vi "DataMatrix AutoDetect Parameters.vi"(7 "_Barcode Type":u16(ring) caption="Barcode Type" items=["Data Matrix", "PDF417", "QR Code"], 8 "error in (no error)":errorcluster, 10 "ROI Descriptor":T20 {"Contours"."Type" items=["No Selection", "Point", "Line", "Rectangle", "Oval", "Polygon", "Free", "Annulus", "Unused2", "Unused3", "Broken Line", "Free Hand Line", "Rotated Rectangle"]}, 11 "Image":T17) -> (0 "error out":errorcluster, 2 "QR Code Auto Detect Values":T8={"QR Search Options"={"Rotation Mode"=enum."Unlimited", "Skip Location?"=FALSE, "Edge Threshold"=30, "Demodulation Mode"=-2, "Cell Sample Size"=-2, "Cell Filter Mode"=-2, "Skew Degrees Allowed"=5}, "QR Description Options"={"Matrix Size (cells)"=0, "Barcode Polarity"=-2, "Mirror Mode"=-2, "QR Model"=0}, "QR Code Cell Size (pixels)"={"Minimum Size"=3, "Maximum Size"=7}} {"QR Description Options"."Mirror Mode" items=["Auto-detect"=-2, "Normal"=0, "Mirrored"=1]; "QR Description Options"."Matrix Size (cells)" items=["Auto-detect"=0, "11x11 - Version 1 (Micro QR Only)"=11, "13x13 - Version 2 (Micro QR Only)"=13, "15x15 - Version 3 (Micro QR Only)"=15, "17x17 - Version 4 (Micro QR Only)"=17, "21x21 - Version 1"=21, "25x25 - Version 2"=25, "29x29 - Version 3"=29, "33x33 - Version 4"=33, "37x37 - Version 5"=37, "41x41 - Version 6"=41, "45x45 - Version 7"=45, "49x49 - Version 8"=49, "53x53 - Version 9"=53, "57x57 - Version 10"=57, "61x61 - Version 11"=61, "65x65 - Version 12"=65, "69x69 - Version 13"=69, "73x73 - Version 14"=73, "77x77 - Version 15"=77, "81x81 - Version 16"=81, "85x85 - Version 17"=85, "89x89 - Version 18"=89, "93x93 - Version 19"=93, "97x97 - Version 20"=97, "101x101 - Version 21"=101, "105x105 - Version 22"=105, "109x109 - Version 23"=109, "113x113 - Version 24"=113, "117x117 - Version 25"=117, "121x121 - Version 26"=121, "125x125 - Version 27"=125, "129x129 - Version 28"=129, "133x133 - Version 29"=133, "137x137 - Version 30"=137, "141x141 - Version 31"=141, "145x145 - Version 32"=145, "149x149 - Version 33"=149, "153x153 - Version 34"=153, "157x157 - Version 35"=157, "161x161 - Version 36"=161, "165x165 - Version 37"=165, "169x169 -  Version 38"=169, "173x173 - Version 39"=173, "177x177 - Version 40"=177]; "QR Description Options"."QR Model" items=["Auto-detect", "Micro", "Model 1", "Model 2"]; "QR Description Options"."Barcode Polarity" items=["Auto-detect"=-2, "Black on White"=0, "White on Black"=1]; "QR Search Options"."Cell Filter Mode" items=["Auto-detect"=-2, "Average"=0, "Median"=1, "Central Average"=2, "High Average"=3, "Low Average"=4, "Very High Average"=5, "Very Low Average"=6, "All Filters"=8]; "QR Search Options"."Cell Sample Size" items=["Auto-detect"=-2, "1x1"=1, "2x2"=2, "3x3"=3, "4x4"=4, "5x5"=5, "6x6"=6, "7x7"=7]; "QR Search Options"."Demodulation Mode" items=["Auto-detect"=-2, "Histogram"=0, "Local Contrast"=1, "Combination"=2, "All"=3]}, 3 "Data Matrix Auto Detect Values Out":T16={"Data Matrix Description Options"={"Aspect Ratio"=0.0, "Rows"=0, "Columns"=0, "Rectangle"=FALSE, "ECC"=-2, "Barcode Polarity"=-2, "Cell Fill Percentage"=-2, "Minimum Border Integrity %"=80.0, "Mirror Mode"=-2}, "Data Matrix Search Options"={"Rotation Mode"=enum."Unlimited", "Skip Location?"=FALSE, "Edge Threshold"=30, "Demodulation Mode"=-2, "Cell Sample Size"=-2, "Cell Filter Mode"=-2, "Skew Degrees Allowed"=5, "Maximum Iterations"=500, "Initial Search Vector Width"=5}, "Data Matrix Size Options"={"Data Matrix Size"={"Minimum Size"=0, "Maximum Size"=0}, "Quiet Zone Width"=10}, "Advanced Options"=[]} {"Advanced Options"."Value" format="%.2f"; "Data Matrix Search Options"."Cell Filter Mode" items=["Auto-detect"=-2, "Average"=0, "Median"=1, "Central Average"=2, "High Average"=3, "Low Average"=4, "Very High Average"=5, "Very Low Average"=6, "All Filters"=8]; "Data Matrix Search Options"."Cell Sample Size" items=["Auto-detect"=-2, "1x1"=1, "2x2"=2, "3x3"=3, "4x4"=4, "5x5"=5, "6x6"=6, "7x7"=7]; "Data Matrix Search Options"."Demodulation Mode" items=["Auto-detect"=-2, "Histogram"=0, "Local Contrast"=1, "Combination"=2, "All"=3]; "Data Matrix Description Options"."Mirror Mode" items=["Auto-detect"=-2, "Normal"=0, "Mirrored"=1]; "Data Matrix Description Options"."ECC" items=["Auto-detect"=-2, "ECC 000"=0, "ECC 050"=50, "ECC 080"=80, "ECC 100"=100, "ECC 140"=140, "ECC 000-140"=190, "ECC 200"=200]; "Data Matrix Description Options"."Minimum Border Integrity %" format="%.2f"; "Data Matrix Description Options"."Aspect Ratio" format="%.2f"; "Data Matrix Description Options"."Cell Fill Percentage" items=["Auto-detect"=-2, "< 30%"=0, ">= 30%"=1]; "Data Matrix Description Options"."Barcode Polarity" items=["Auto-detect"=-2, "Black on White"=0, "White on Black"=1]})   [LabVIEW 2015]
uses:
  <vilib>/vision/Instrument.llb/Data Matrix Description Options.ctl
  <vilib>/vision/Instrument.llb/ECC Type.ctl
  <vilib>/vision/Instrument.llb/Data Matrix Polarity.ctl
  <vilib>/vision/Instrument.llb/Cell Fill Percentage.ctl
  <vilib>/vision/Instrument.llb/Data Matrix Mirror.ctl
  <vilib>/vision/Instrument.llb/Data Matrix Search Options.ctl
  <vilib>/vision/Instrument.llb/Demodulation Mode.ctl
  <vilib>/vision/Instrument.llb/Cell Sample Size.ctl
  <vilib>/vision/Instrument.llb/Cell Filter Mode.ctl
  <vilib>/vision/Instrument.llb/Data Matrix Size Options.ctl
  <vilib>/vision/Instrument.llb/Data Matrix Advanced Options.ctl
  <vilib>/vision/Instrument.llb/QR Code Search Options.ctl
  <vilib>/vision/Instrument.llb/QR Code Description Options.ctl
  <vilib>/vision/Instrument.llb/QR Code Model Type.ctl
  <vilib>/vision/Image Controls.llb/IMAQ Image.ctl
  <vilib>/vision/NI_Vision_Development_Module.lvlib
panel:
  in  "QR Code Auto Detect Values":T18(array[cluster])=[{"QR Search Options"={"Rotation Mode"=enum."Unlimited", "Skip Location?"=FALSE, "Edge Threshold"=30, "Demodulation Mode"=-2, "Cell Sample Size"=-2, "Cell Filter Mode"=2, "Skew Degrees Allowed"=5}, "QR Description Options"={"Matrix Size (cells)"=0, "Barcode Polarity"=-2, "Mirror Mode"=-2, "QR Model"=0}, "QR Code Cell Size (pixels)"={"Minimum Size"=3, "Maximum Size"=15}}, {"QR Search Options"={"Rotation Mode"=enum."Unlimited", "Skip Location?"=FALSE, "Edge Threshold"=15, "Demodulation Mode"=-2, "Cell Sample Size"=-2, "Cell Filter Mode"=2, "Skew Degrees Allowed"=15}, "QR Description Options"={"Matrix Size (cells)"=0, "Barcode Polarity"=-2, "Mirror Mode"=0, "QR Model"=0}, "QR Code Cell Size (pixels)"={"Minimum Size"=3, "Maximum Size"=15}}, {"QR Search Options"={"Rotation Mode"=enum."Unlimited", "Skip Location?"=FALSE, "Edge Threshold"=15, "Demodulation Mode"=-2, "Cell Sample Size"=-2, "Cell Filter Mode"=2, "Skew Degrees Allowed"=15}, "QR Description Options"={"Matrix Size (cells)"=0, "Barcode Polarity"=-2, "Mirror Mode"=-2, "QR Model"=0}, "QR Code Cell Size (pixels)"={"Minimum Size"=3, "Maximum Size"=15}}, {"QR Search Options"={"Rotation Mode"=enum."Unlimited", "Skip Location?"=FALSE, "Edge Threshold"=5, "Demodulation Mode"=-2, "Cell Sample Size"=-2, "Cell Filter Mode"=2, "Skew Degrees Allowed"=15}, "QR Description Options"={"Matrix Size (cells)"=0, "Barcode Polarity"=-2, "Mirror Mode"=-2, "QR Model"=0}, "QR Code Cell Size (pixels)"={"Minimum Size"=3, "Maximum Size"=15}}, {"QR Search Options"={"Rotation Mode"=enum."Unlimited", "Skip Location?"=FALSE, "Edge Threshold"=30, "Demodulation Mode"=-2, "Cell Sample Size"=-2, "Cell Filter Mode"=-2, "Skew Degrees Allowed"=3}, "QR Description Options"={"Matrix Size (cells)"=0, "Barcode Polarity"=-2, "Mirror Mode"=-2, "QR Model"=0}, "QR Code Cell Size (pixels)"={"Minimum Size"=3, "Maximum Size"=15}}, {"QR Search Options"={"Rotation Mode"=enum."Unlimited", "Skip Location?"=FALSE, "Edge Threshold"=5, "Demodulation Mode"=-2, "Cell Sample Size"=-2, "Cell Filter Mode"=2, "Skew Degrees Allowed"=5}, "QR Description Options"={"Matrix Size (cells)"=0, "Barcode Polarity"=-2, "Mirror Mode"=-2, "QR Model"=0}, "QR Code Cell Size (pixels)"={"Minimum Size"=3, "Maximum Size"=15}}, {"QR Search Options"={"Rotation Mode"=enum."Unlimited", "Skip Location?"=FALSE, "Edge Threshold"=20, "Demodulation Mode"=-2, "Cell Sample Size"=-2, "Cell Filter Mode"=2, "Skew Degrees Allowed"=5}, "QR Description Options"={"Matrix Size (cells)"=0, "Barcode Polarity"=-2, "Mirror Mode"=-2, "QR Model"=0}, "QR Code Cell Size (pixels)"={"Minimum Size"=3, "Maximum Size"=15}}, {"QR Search Options"={"Rotation Mode"=enum."Unlimited", "Skip Location?"=FALSE, "Edge Threshold"=50, "Demodulation Mode"=-2, "Cell Sample Size"=-2, "Cell Filter Mode"=2, "Skew Degrees Allowed"=5}, "QR Description Options"={"Matrix Size (cells)"=0, "Barcode Polarity"=-2, "Mirror Mode"=-2, "QR Model"=0}, "QR Code Cell Size (pixels)"={"Minimum Size"=3, "Maximum Size"=15}}] {"QR Description Options"."Mirror Mode" items=["Auto-detect"=-2, "Normal"=0, "Mirrored"=1]; "QR Description Options"."Matrix Size (cells)" items=["Auto-detect"=0, "11x11 - Version 1 (Micro QR Only)"=11, "13x13 - Version 2 (Micro QR Only)"=13, "15x15 - Version 3 (Micro QR Only)"=15, "17x17 - Version 4 (Micro QR Only)"=17, "21x21 - Version 1"=21, "25x25 - Version 2"=25, "29x29 - Version 3"=29, "33x33 - Version 4"=33, "37x37 - Version 5"=37, "41x41 - Version 6"=41, "45x45 - Version 7"=45, "49x49 - Version 8"=49, "53x53 - Version 9"=53, "57x57 - Version 10"=57, "61x61 - Version 11"=61, "65x65 - Version 12"=65, "69x69 - Version 13"=69, "73x73 - Version 14"=73, "77x77 - Version 15"=77, "81x81 - Version 16"=81, "85x85 - Version 17"=85, "89x89 - Version 18"=89, "93x93 - Version 19"=93, "97x97 - Version 20"=97, "101x101 - Version 21"=101, "105x105 - Version 22"=105, "109x109 - Version 23"=109, "113x113 - Version 24"=113, "117x117 - Version 25"=117, "121x121 - Version 26"=121, "125x125 - Version 27"=125, "129x129 - Version 28"=129, "133x133 - Version 29"=133, "137x137 - Version 30"=137, "141x141 - Version 31"=141, "145x145 - Version 32"=145, "149x149 - Version 33"=149, "153x153 - Version 34"=153, "157x157 - Version 35"=157, "161x161 - Version 36"=161, "165x165 - Version 37"=165, "169x169 -  Version 38"=169, "173x173 - Version 39"=173, "177x177 - Version 40"=177]; "QR Description Options"."QR Model" items=["Auto-detect", "Micro", "Model 1", "Model 2"]; "QR Description Options"."Barcode Polarity" items=["Auto-detect"=-2, "Black on White"=0, "White on Black"=1]; "QR Search Options"."Cell Filter Mode" items=["Auto-detect"=-2, "Average"=0, "Median"=1, "Central Average"=2, "High Average"=3, "Low Average"=4, "Very High Average"=5, "Very Low Average"=6, "All Filters"=8]; "QR Search Options"."Cell Sample Size" items=["Auto-detect"=-2, "1x1"=1, "2x2"=2, "3x3"=3, "4x4"=4, "5x5"=5, "6x6"=6, "7x7"=7]; "QR Search Options"."Demodulation Mode" items=["Auto-detect"=-2, "Histogram"=0, "Local Contrast"=1, "Combination"=2, "All"=3]}
  in  "Data Matrix Auto Detect Values":T19(array[cluster])=[{"Data Matrix Description Options"={"Aspect Ratio"=0.0, "Rows"=0, "Columns"=0, "Rectangle"=FALSE, "ECC"=-2, "Barcode Polarity"=-2, "Cell Fill Percentage"=-2, "Minimum Border Integrity %"=80.0, "Mirror Mode"=-2}, "Data Matrix Search Options"={"Rotation Mode"=enum."Unlimited", "Skip Location?"=FALSE, "Edge Threshold"=30, "Demodulation Mode"=-2, "Cell Sample Size"=-2, "Cell Filter Mode"=2, "Skew Degrees Allowed"=5, "Maximum Iterations"=100, "Initial Search Vector Width"=5}, "Data Matrix Size Options"={"Data Matrix Size"={"Minimum Size"=0, "Maximum Size"=0}, "Quiet Zone Width"=0}, "Advanced Options"=[]}, {"Data Matrix Description Options"={"Aspect Ratio"=0.0, "Rows"=0, "Columns"=0, "Rectangle"=FALSE, "ECC"=-2, "Barcode Polarity"=-2, "Cell Fill Percentage"=-2, "Minimum Border Integrity %"=80.0, "Mirror Mode"=-2}, "Data Matrix Search Options"={"Rotation Mode"=enum."Unlimited", "Skip Location?"=FALSE, "Edge Threshold"=30, "Demodulation Mode"=-2, "Cell Sample Size"=-2, "Cell Filter Mode"=2, "Skew Degrees Allowed"=5, "Maximum Iterations"=100, "Initial Search Vector Width"=15}, "Data Matrix Size Options"={"Data Matrix Size"={"Minimum Size"=0, "Maximum Size"=0}, "Quiet Zone Width"=0}, "Advanced Options"=[{"Option"=enum."Line Detection", " Value"=1.0}]}, {"Data Matrix Description Options"={"Aspect Ratio"=0.0, "Rows"=0, "Columns"=0, "Rectangle"=FALSE, "ECC"=-2, "Barcode Polarity"=-2, "Cell Fill Percentage"=-2, "Minimum Border Integrity %"=75.0, "Mirror Mode"=0}, "Data Matrix Search Options"={"Rotation Mode"=enum."Unlimited", "Skip Location?"=FALSE, "Edge Threshold"=15, "Demodulation Mode"=-2, "Cell Sample Size"=-2, "Cell Filter Mode"=2, "Skew Degrees Allowed"=15, "Maximum Iterations"=500, "Initial Search Vector Width"=15}, "Data Matrix Size Options"={"Data Matrix Size"={"Minimum Size"=0, "Maximum Size"=0}, "Quiet Zone Width"=0}, "Advanced Options"=[]}, {"Data Matrix Description Options"={"Aspect Ratio"=0.0, "Rows"=0, "Columns"=0, "Rectangle"=FALSE, "ECC"=-2, "Barcode Polarity"=-2, "Cell Fill Percentage"=-2, "Minimum Border Integrity %"=75.0, "Mirror Mode"=-2}, "Data Matrix Search Options"={"Rotation Mode"=enum."Unlimited", "Skip Location?"=FALSE, "Edge Threshold"=15, "Demodulation Mode"=-2, "Cell Sample Size"=-2, "Cell Filter Mode"=2, "Skew Degrees Allowed"=15, "Maximum Iterations"=100, "Initial Search Vector Width"=15}, "Data Matrix Size Options"={"Data Matrix Size"={"Minimum Size"=0, "Maximum Size"=0}, "Quiet Zone Width"=0}, "Advanced Options"=[{"Option"=enum."Line Detection", " Value"=1.0}, {"Option"=enum."HighLight Filter", " Value"=0.0}]}, {"Data Matrix Description Options"={"Aspect Ratio"=0.0, "Rows"=0, "Columns"=0, "Rectangle"=FALSE, "ECC"=-2, "Barcode Polarity"=-2, "Cell Fill Percentage"=-2, "Minimum Border Integrity %"=75.0, "Mirror Mode"=-2}, "Data Matrix Search Options"={"Rotation Mode"=enum."Unlimited", "Skip Location?"=FALSE, "Edge Threshold"=5, "Demodulation Mode"=-2, "Cell Sample Size"=-2, "Cell Filter Mode"=2, "Skew Degrees Allowed"=15, "Maximum Iterations"=100, "Initial Search Vector Width"=15}, "Data Matrix Size Options"={"Data Matrix Size"={"Minimum Size"=0, "Maximum Size"=0}, "Quiet Zone Width"=0}, "Advanced Options"=[{"Option"=enum."Line Detection", " Value"=0.0}, {"Option"=enum."HighLight Filter", " Value"=0.0}]}, {"Data Matrix Description Options"={"Aspect Ratio"=0.0, "Rows"=0, "Columns"=0, "Rectangle"=FALSE, "ECC"=-2, "Barcode Polarity"=-2, "Cell Fill Percentage"=-2, "Minimum Border Integrity %"=75.0, "Mirror Mode"=-2}, "Data Matrix Search Options"={"Rotation Mode"=enum."Unlimited", "Skip Location?"=FALSE, "Edge Threshold"=5, "Demodulation Mode"=-2, "Cell Sample Size"=-2, "Cell Filter Mode"=2, "Skew Degrees Allowed"=15, "Maximum Iterations"=100, "Initial Search Vector Width"=15}, "Data Matrix Size Options"={"Data Matrix Size"={"Minimum Size"=0, "Maximum Size"=0}, "Quiet Zone Width"=0}, "Advanced Options"=[{"Option"=enum."Line Detection", " Value"=1.0}, {"Option"=enum."HighLight Filter", " Value"=1.0}]}, {"Data Matrix Description Options"={"Aspect Ratio"=0.0, "Rows"=0, "Columns"=0, "Rectangle"=FALSE, "ECC"=-2, "Barcode Polarity"=-2, "Cell Fill Percentage"=-2, "Minimum Border Integrity %"=80.0, "Mirror Mode"=-2}, "Data Matrix Search Options"={"Rotation Mode"=enum."Unlimited", "Skip Location?"=FALSE, "Edge Threshold"=30, "Demodulation Mode"=-2, "Cell Sample Size"=-2, "Cell Filter Mode"=-2, "Skew Degrees Allowed"=3, "Maximum Iterations"=100, "Initial Search Vector Width"=5}, "Data Matrix Size Options"={"Data Matrix Size"={"Minimum Size"=75, "Maximum Size"=175}, "Quiet Zone Width"=0}, "Advanced Options"=[{"Option"=enum."Line Detection", " Value"=0.0}, {"Option"=enum."HighLight Filter", " Value"=0.0}]}, {"Data Matrix Description Options"={"Aspect Ratio"=0.0, "Rows"=0, "Columns"=0, "Rectangle"=FALSE, "ECC"=-2, "Barcode Polarity"=-2, "Cell Fill Percentage"=-2, "Minimum Border Integrity %"=80.0, "Mirror Mode"=-2}, "Data Matrix Search Options"={"Rotation Mode"=enum."Unlimited", "Skip Location?"=FALSE, "Edge Threshold"=5, "Demodulation Mode"=-2, "Cell Sample Size"=-2, "Cell Filter Mode"=2, "Skew Degrees Allowed"=5, "Maximum Iterations"=100, "Initial Search Vector Width"=5}, "Data Matrix Size Options"={"Data Matrix Size"={"Minimum Size"=75, "Maximum Size"=175}, "Quiet Zone Width"=0}, "Advanced Options"=[]}, {"Data Matrix Description Options"={"Aspect Ratio"=0.0, "Rows"=0, "Columns"=0, "Rectangle"=FALSE, "ECC"=-2, "Barcode Polarity"=-2, "Cell Fill Percentage"=-2, "Minimum Border Integrity %"=80.0, "Mirror Mode"=-2}, "Data Matrix Search Options"={"Rotation Mode"=enum."Unlimited", "Skip Location?"=FALSE, "Edge Threshold"=20, "Demodulation Mode"=-2, "Cell Sample Size"=-2, "Cell Filter Mode"=2, "Skew Degrees Allowed"=5, "Maximum Iterations"=100, "Initial Search Vector Width"=5}, "Data Matrix Size Options"={"Data Matrix Size"={"Minimum Size"=0, "Maximum Size"=0}, "Quiet Zone Width"=0}, "Advanced Options"=[{"Option"=enum."Refine Bounding Box", " Value"=0.0}]}, {"Data Matrix Description Options"={"Aspect Ratio"=0.0, "Rows"=0, "Columns"=0, "Rectangle"=FALSE, "ECC"=-2, "Barcode Polarity"=-2, "Cell Fill Percentage"=-2, "Minimum Border Integrity %"=80.0, "Mirror Mode"=-2}, "Data Matrix Search Options"={"Rotation Mode"=enum."Unlimited", "Skip Location?"=FALSE, "Edge Threshold"=20, "Demodulation Mode"=-2, "Cell Sample Size"=-2, "Cell Filter Mode"=2, "Skew Degrees Allowed"=5, "Maximum Iterations"=50, "Initial Search Vector Width"=15}, "Data Matrix Size Options"={"Data Matrix Size"={"Minimum Size"=0, "Maximum Size"=0}, "Quiet Zone Width"=0}, "Advanced Options"=[{"Option"=enum."Line Detection", " Value"=1.0}]}, {"Data Matrix Description Options"={"Aspect Ratio"=0.0, "Rows"=0, "Columns"=0, "Rectangle"=FALSE, "ECC"=-2, "Barcode Polarity"=-2, "Cell Fill Percentage"=-2, "Minimum Border Integrity %"=80.0, "Mirror Mode"=-2}, "Data Matrix Search Options"={"Rotation Mode"=enum."Unlimited", "Skip Location?"=FALSE, "Edge Threshold"=50, "Demodulation Mode"=-2, "Cell Sample Size"=-2, "Cell Filter Mode"=2, "Skew Degrees Allowed"=5, "Maximum Iterations"=50, "Initial Search Vector Width"=5}, "Data Matrix Size Options"={"Data Matrix Size"={"Minimum Size"=50, "Maximum Size"=300}, "Quiet Zone Width"=0}, "Advanced Options"=[{"Option"=enum."Line Detection", " Value"=0.0}]}, {"Data Matrix Description Options"={"Aspect Ratio"=0.0, "Rows"=0, "Columns"=0, "Rectangle"=FALSE, "ECC"=-2, "Barcode Polarity"=-2, "Cell Fill Percentage"=-2, "Minimum Border Integrity %"=80.0, "Mirror Mode"=-2}, "Data Matrix Search Options"={"Rotation Mode"=enum."Unlimited", "Skip Location?"=FALSE, "Edge Threshold"=30, "Demodulation Mode"=-2, "Cell Sample Size"=-2, "Cell Filter Mode"=2, "Skew Degrees Allowed"=5, "Maximum Iterations"=50, "Initial Search Vector Width"=5}, "Data Matrix Size Options"={"Data Matrix Size"={"Minimum Size"=175, "Maximum Size"=350}, "Quiet Zone Width"=0}, "Advanced Options"=[{"Option"=enum."Refine Bounding Box", " Value"=1.0}]}, {"Data Matrix Description Options"={"Aspect Ratio"=0.0, "Rows"=0, "Columns"=0, "Rectangle"=TRUE, "ECC"=-2, "Barcode Polarity"=-2, "Cell Fill Percentage"=-2, "Minimum Border Integrity %"=80.0, "Mirror Mode"=-2}, "Data Matrix Search Options"={"Rotation Mode"=enum."Unlimited", "Skip Location?"=FALSE, "Edge Threshold"=30, "Demodulation Mode"=-2, "Cell Sample Size"=-2, "Cell Filter Mode"=2, "Skew Degrees Allowed"=5, "Maximum Iterations"=30, "Initial Search Vector Width"=5}, "Data Matrix Size Options"={"Data Matrix Size"={"Minimum Size"=0, "Maximum Size"=0}, "Quiet Zone Width"=0}, "Advanced Options"=[{"Option"=enum."Line Detection", " Value"=1.0}]}] {"Advanced Options"."Value" format="%.2f"; "Data Matrix Search Options"."Cell Filter Mode" items=["Auto-detect"=-2, "Average"=0, "Median"=1, "Central Average"=2, "High Average"=3, "Low Average"=4, "Very High Average"=5, "Very Low Average"=6, "All Filters"=8]; "Data Matrix Search Options"."Cell Sample Size" items=["Auto-detect"=-2, "1x1"=1, "2x2"=2, "3x3"=3, "4x4"=4, "5x5"=5, "6x6"=6, "7x7"=7]; "Data Matrix Search Options"."Demodulation Mode" items=["Auto-detect"=-2, "Histogram"=0, "Local Contrast"=1, "Combination"=2, "All"=3]; "Data Matrix Description Options"."Mirror Mode" items=["Auto-detect"=-2, "Normal"=0, "Mirrored"=1]; "Data Matrix Description Options"."ECC" items=["Auto-detect"=-2, "ECC 000"=0, "ECC 050"=50, "ECC 080"=80, "ECC 100"=100, "ECC 140"=140, "ECC 000-140"=190, "ECC 200"=200]; "Data Matrix Description Options"."Minimum Border Integrity %" format="%.2f"; "Data Matrix Description Options"."Aspect Ratio" format="%.2f"; "Data Matrix Description Options"."Cell Fill Percentage" items=["Auto-detect"=-2, "< 30%"=0, ">= 30%"=1]; "Data Matrix Description Options"."Barcode Polarity" items=["Auto-detect"=-2, "Black on White"=0, "White on Black"=1]}
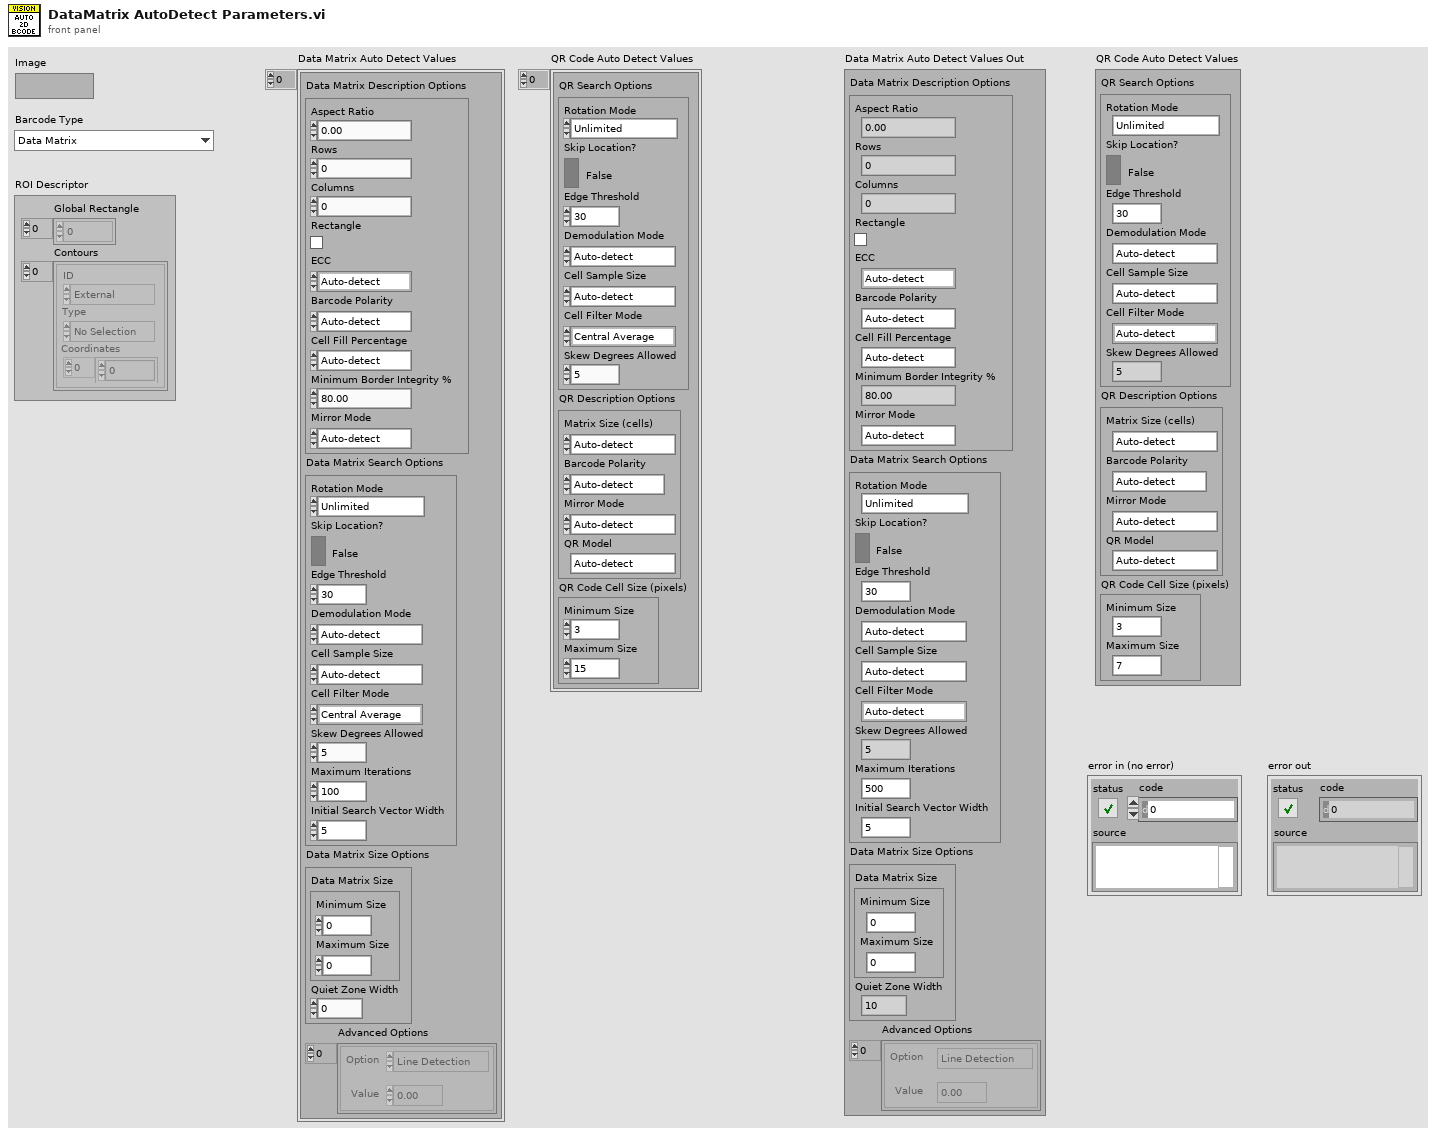
[diagram p1: front panel]
types:
  T1 = typedef "QR Code Search Options.ctl" = cluster{"Rotation Mode":enum32{"Unlimited", "0 Degrees", "90 Degrees", "180 Degrees", "270 Degrees"}, "Skip Location?":bool, "Edge Threshold":u32, "Demodulation Mode":T2, "Cell Sample Size":T3, "Cell Filter Mode":T4, "Skew Degrees Allowed":u32}
  T2 = typedef "Demodulation Mode.ctl" = i32
  T3 = typedef "Cell Sample Size.ctl" = i32
  T4 = typedef "Cell Filter Mode.ctl" = i32
  T5 = typedef "QR Code Description Options.ctl" = cluster{"Matrix Size (cells)":i32, "Barcode Polarity":T6, "Mirror Mode":i32, "QR Model":T7}
  T6 = typedef "Data Matrix Polarity.ctl" = i32
  T7 = typedef "QR Code Model Type.ctl" = i32
  T8 = cluster{"QR Search Options":T1, "QR Description Options":T5, "QR Code Cell Size (pixels)":cluster{"Minimum Size":u32, "Maximum Size":u32}}
  T9 = typedef "Data Matrix Description Options.ctl" = cluster{"Aspect Ratio":sgl, "Rows":u32, "Columns":u32, "Rectangle":bool, "ECC":T10, "Barcode Polarity":T6, "Cell Fill Percentage":T11, "Minimum Border Integrity %":sgl, "Mirror Mode":T12}
  T10 = typedef "ECC Type.ctl" = i32
  T11 = typedef "Cell Fill Percentage.ctl" = i32
  T12 = typedef "Data Matrix Mirror.ctl" = i32
  T13 = typedef "Data Matrix Search Options.ctl" = cluster{"Rotation Mode":enum32{"Unlimited", "0 Degrees", "90 Degrees", "180 Degrees", "270 Degrees"}, "Skip Location?":bool, "Edge Threshold":u32, "Demodulation Mode":T2, "Cell Sample Size":T3, "Cell Filter Mode":T4, "Skew Degrees Allowed":u32, "Maximum Iterations":u32, "Initial Search Vector Width":u32}
  T14 = typedef "Data Matrix Size Options.ctl" = cluster{"Data Matrix Size":cluster{"Minimum Size":u32, "Maximum Size":u32}, "Quiet Zone Width":u32}
  T15 = typedef "Data Matrix Advanced Options.ctl" = cluster{"Option":enum32{"Line Detection", "HighLight Filter", "Aggressive", "FNC1", "Refine Bounding Box"}, " Value":dbl}
  T16 = cluster{"Data Matrix Description Options":T9, "Data Matrix Search Options":T13, "Data Matrix Size Options":T14, "Advanced Options":T15[]}
  T17 = typedef "IMAQ Image.ctl" = refnum<image>
  T18 = cluster{"QR Search Options":T1, "QR Description Options":T5, "QR Code Cell Size (pixels)":cluster{"Minimum Size":u32, "Maximum Size":u32}}[]
  T19 = cluster{"Data Matrix Description Options":T9, "Data Matrix Search Options":T13, "Data Matrix Size Options":T14, "Advanced Options":T15[]}[]
  T20 = cluster{"Global Rectangle":i32[], "Contours":cluster{"ID":enum32{"External", "Internal"}, "Type":u32, "Coordinates":i32[]}[]}
  T21 = typedef "Data Matrix Report.ctl" = cluster{"Found?":bool, "Binary?":bool, "Data":string, "Bounding Box":cluster{"x":sgl, "y":sgl}[], "Errors Corrected":u32, "Erasures Corrected":u32, "Aspect Ratio":sgl, "Rows":u32, "Columns":u32, "ECC":T10, "Barcode Polarity":T6, "Cell Fill Percentage":T11, "Border Integrity":sgl, "Mirrored?":bool, "Minimum Edge Strength":u32, "Demodulation Mode":T2, "Cell Sample Size":T3, "Cell Filter Mode":T4, "Iterations":u32}
  T22 = typedef "QR Code Report.ctl" = cluster{"Found?":bool, "Data":string, "Bounding Box":cluster{"x":sgl, "y":sgl}[], "Errors Corrected":u32, "Dimensions (Rows/Cols)":u32, "Version":u32, "QR Model":T7, "Stream Mode":T23, "Barcode Polarity":T6, "Mirrored?":bool, "Append Stream Position":u32, "Size of Append Stream":u32, "First EAN-128 ID":i32, "First Alternate Language ID":i32, "Append Stream ID":u32, "Minimum Edge Strength":u32, "Demodulation Mode":T2, "Cell Sample Size":T3, "Cell Filter Mode":T4}
  T23 = typedef "QR Code Stream Mode Type.ctl" = i32
  T24 = enum32{"Line Detection", "HighLight Filter", "Aggressive", "FNC1", "Refine Bounding Box"}[]
  T25 = enum32{"Line Detection", "HighLight Filter", "Aggressive", "FNC1", "Refine Bounding Box"}
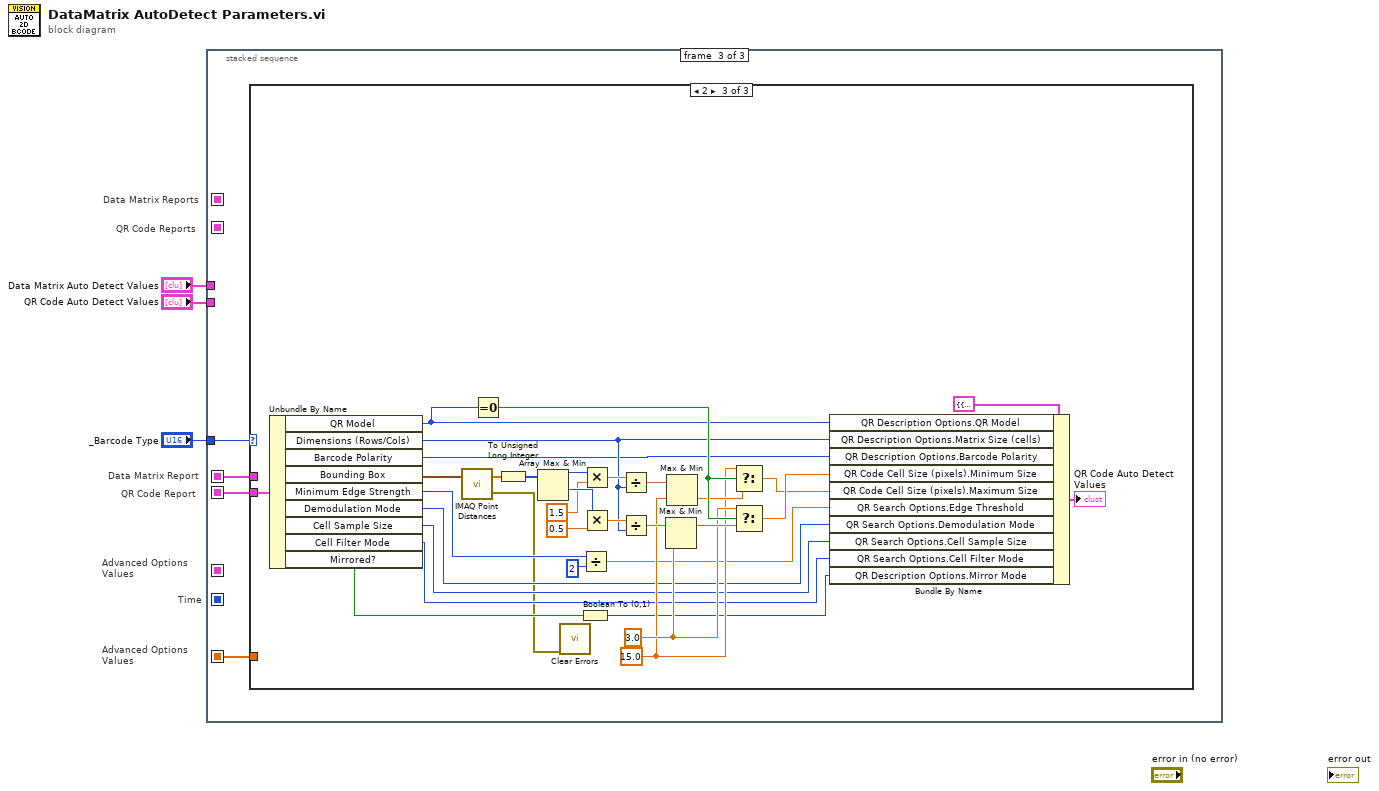
[diagram p0: block diagram]
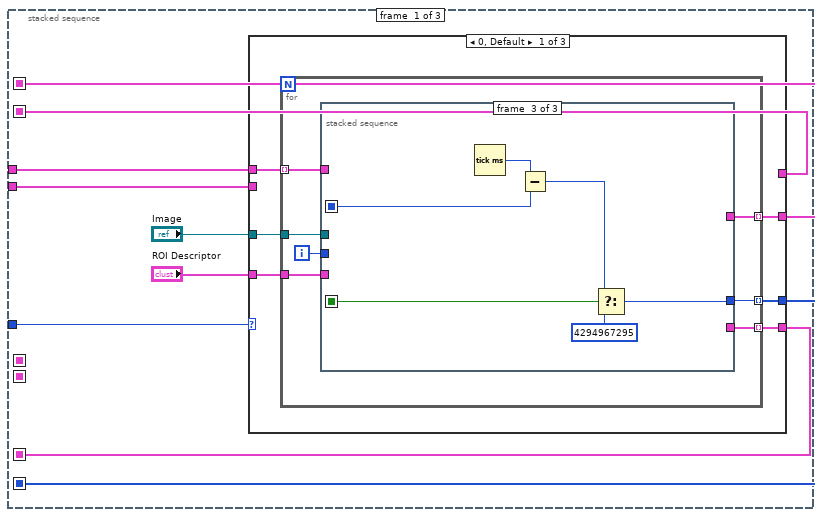
[diagram p2: hidden frame]
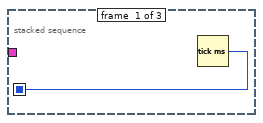
[diagram p3: hidden frame]
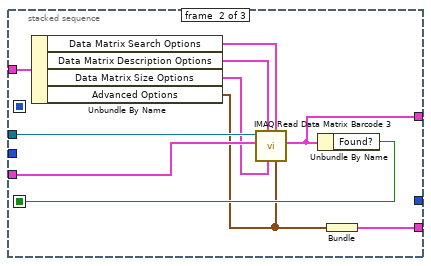
[diagram p4: hidden frame]
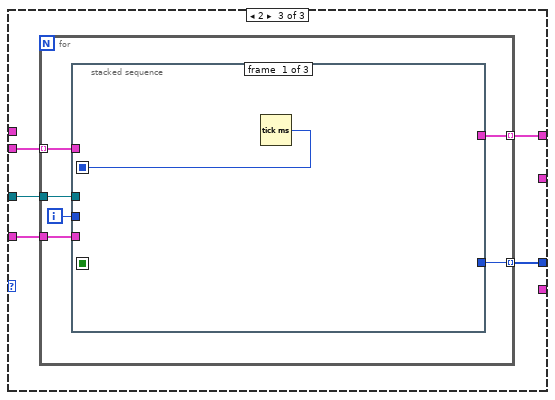
[diagram p6: hidden frame]
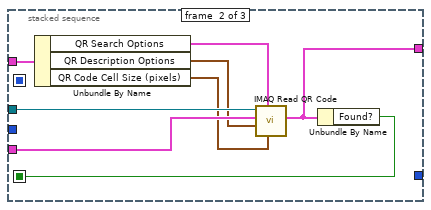
[diagram p7: hidden frame]
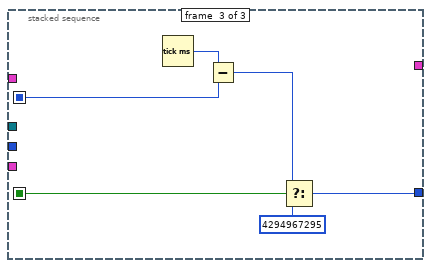
[diagram p8: hidden frame]
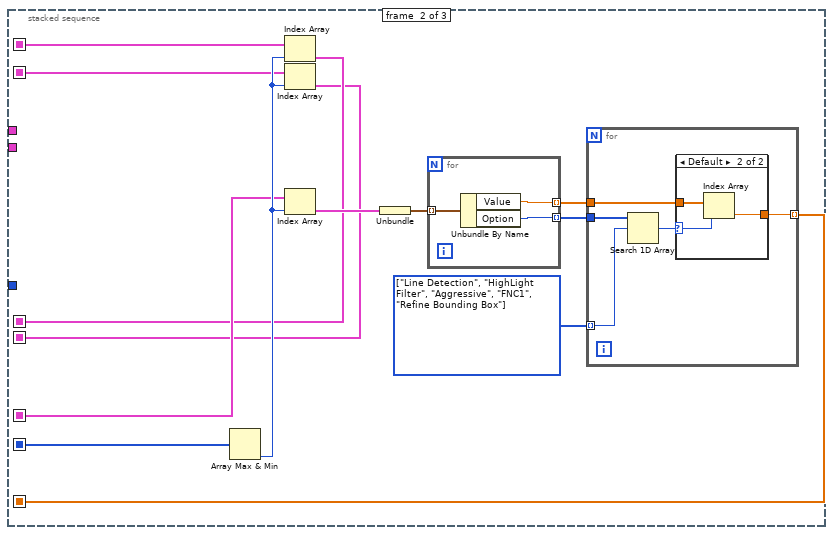
[diagram p9: hidden frame]
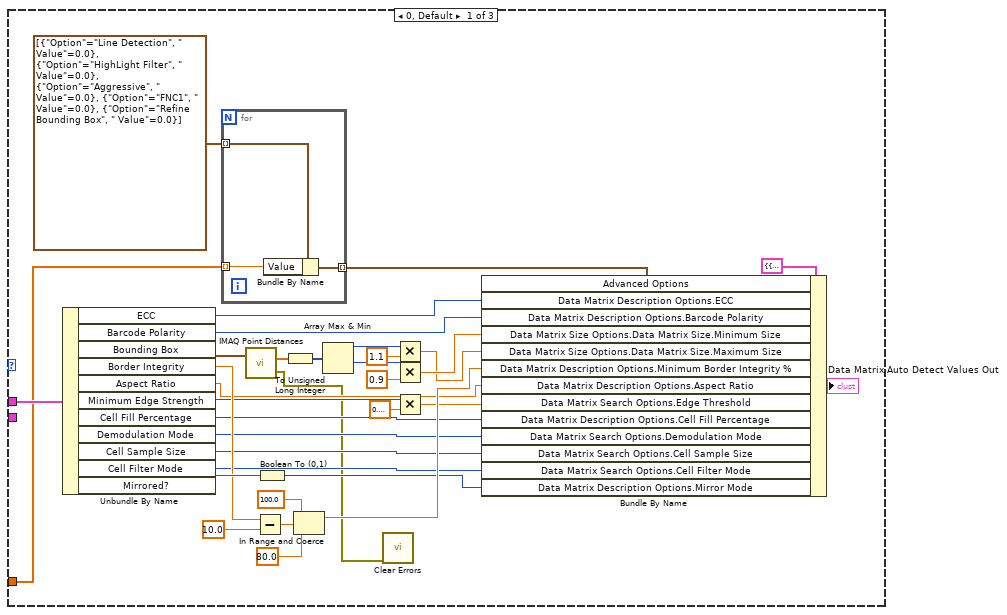
[diagram p11: hidden frame]
diagram:
  # "QR Code Reports"
  # "Data Matrix Reports"
  # "Time"
  # "Advanced Options\nValues"
  # "Advanced Options\nValues"
  # "QR Code Report"
  # "Data Matrix Report"
  n1 = stacked-sequence {
    seq-local: [_ w70 _] -> [_ _ w96]
    seq-local: [_ w69 _] -> [_ _ w95]
    seq-local: [w11 _ _] -> [_ w72 _]
    seq-local: [_ w78 _] -> [_ _ w94]
    seq-local: [w9 _ _] -> [_ w73 _]
    seq-local: [w10 _ _] -> [_ w75 _]
    seq-local: [w8 _ _] -> [_ w74 _]
    tunnel: "_Barcode Type" -> [w12 _ w93]
    tunnel: "Data Matrix Auto Detect Values" -> [w7 _ _]
    tunnel: "QR Code Auto Detect Values" -> [w6 _ _]
    frame #0 {
      n2 = case shown="0, Default" w12 {
        tunnel: "Image" -> [w18 _ w47]
        tunnel: "ROI Descriptor" -> [w17 _ w46]
        tunnel: [w16 _ w45] -> w10
        tunnel: [w15 _ _] -> w8
        tunnel: [_ _ w44] -> w9
        tunnel: [w14 _ _] -> w11
        tunnel: w7 -> [w13 _ _]
        tunnel: w6 -> [_ _ w43]
        frame 0, Default {
          n3 = for {
            tunnel: w13 -> [w25] mode=indexing
            tunnel: w18 -> [w24]
            tunnel: w17 -> [w23]
            tunnel: [w22] -> w15 mode=indexing
            tunnel: [w21] -> w16 mode=indexing
            tunnel: [w20] -> w14 mode=indexing
            i -> [w19]
            n4 = stacked-sequence {
              seq-local: [w26 _ _] -> [_ _ w41]
              seq-local: [_ w32 _] -> [_ _ w40]
              tunnel: w25 -> [_ w34 _]
              tunnel: w24 -> [_ w36 _]
              tunnel: w23 -> [_ w35 _]
              tunnel: [_ w33 _] -> w22
              tunnel: [_ _ w37] -> w21
              tunnel: [_ w31 _] -> w20
              tunnel: w19 -> [_ _ _]
              frame #0 {
                n5 = Tick Count (ms)() -> (millisecond timer value=w26:u32)
              }
              frame #1 {
                n6 = Unbundle By Name(w34) -> ("Data Matrix Search Options"=w29:T13, "Data Matrix Description Options"=w30:T9, "Data Matrix Size Options"=w28:T14, "Advanced Options"=w27:T15[])
                n7 = call "IMAQ Read Data Matrix Barcode 3"("Advanced Options"=w27, "Data Matrix Search Options"=w29, "Data Matrix Size Options"=w28, "Data Matrix Description Options"=w30, "ROI Descriptor"=w35, "Image"=w36) -> ("Data Matrix Report"=w33:T21)  [unwired: 2 in, 3 out]
                n8 = Unbundle By Name(w33) -> ("Found?"=w32:bool)
                n9 = Bundle("Advanced Options"=w27) -> (w31:cluster{"Advanced Options":T15[]})  [unwired: 1 in]
              }
              frame #2 {
                n10 = Tick Count (ms)() -> (millisecond timer value=w42:u32)
                n11 = Subtract(x=w42, y=w41) -> (x-y=w39:u32)
                n12 = Select(t=w39, s=w40, f=u32 4294967295) -> (s? t:f=w37:u32)
              }
            }
          }
        }
        frame 1 {
        }
        frame 2 {
          n13 = for {
            tunnel: w47 -> [w53]
            tunnel: w46 -> [w52]
            tunnel: [w51] -> w44 mode=indexing
            tunnel: [w50] -> w45 mode=indexing
            tunnel: w43 -> [w49] mode=indexing
            i -> [w48]
            n14 = stacked-sequence {
              seq-local: [w54 _ _] -> [_ _ w67]
              seq-local: [_ w59 _] -> [_ _ w66]
              tunnel: w53 -> [_ w62 _]
              tunnel: w52 -> [_ w61 _]
              tunnel: [_ w60 _] -> w51
              tunnel: [_ _ w63] -> w50
              tunnel: w49 -> [_ w55 _]
              tunnel: w48 -> [_ _ _]
              frame #0 {
                n15 = Tick Count (ms)() -> (millisecond timer value=w54:u32)
              }
              frame #1 {
                n16 = Unbundle By Name(w55) -> ("QR Search Options"=w58:T1, "QR Description Options"=w57:T5, "QR Code Cell Size (pixels)"=w56:cluster{"Minimum Size":u32, "Maximum Size":u32})
                n17 = call "IMAQ Read QR Code"("QR Code Cell Size (pixels)"=w56, "QR Search Options"=w58, "QR Description Options"=w57, "ROI Descriptor"=w61, "Image"=w62) -> ("QR Code Report"=w60:T22)  [unwired: 2 in, 4 out]
                n18 = Unbundle By Name(w60) -> ("Found?"=w59:bool)
              }
              frame #2 {
                n19 = Tick Count (ms)() -> (millisecond timer value=w68:u32)
                n20 = Subtract(x=w68, y=w67) -> (x-y=w65:u32)
                n21 = Select(t=w65, s=w66, f=u32 4294967295) -> (s? t:f=w63:u32)
              }
            }
          }
        }
      }
    }
    frame #1 {
      w81 = T24 [enum."Line Detection", enum."HighLight Filter", enum."Aggressive", enum."FNC1", enum."Refine Bounding Box"] items=["Line Detection", "HighLight Filter", "Aggressive", "FNC1", "Refine Bounding Box"]
      n22 = Array Max & Min(array=w75) -> (min index (indices)=w77:i32)  [unwired: 3 out]
      n23 = Index Array(array=w74, index=w77) -> (element=w70:T21)
      n24 = Index Array(array=w73, index=w77) -> (element=w69:T22)
      n25 = Index Array(array=w72, index=w77) -> (element=w76:cluster{"Advanced Options":T15[]})
      n26 = Unbundle(w76) -> ("Advanced Options"=w71:T15[])
      n27 = for {
        tunnel: w71 -> [w90] mode=indexing
        tunnel: [w92] -> w80 mode=indexing
        tunnel: [w91] -> w79 mode=indexing
        n28 = Unbundle By Name(w90) -> ("Value"=w91:dbl, "Option"=w92:T25)
      }
      n29 = for {
        tunnel: w81 -> [w86] mode=indexing
        tunnel: w80 -> [w85]
        tunnel: w79 -> [w83]
        tunnel: [w82] -> w78 mode=indexing
        n30 = Search 1D Array(1D array=w85, element=w86) -> (index of element=w84:i32)  [unwired: 1 in]
        n31 = case shown="Default" w84 {
          selector: w84 -> [_ w89]
          tunnel: w83 -> [_ w88]
          tunnel: [_ w87] -> w82
          frame -1 {
          }
          frame Default {
            n32 = Index Array(array=w88, index=w89) -> (element=w87:dbl)
          }
        }
      }
    }
    frame #2 {
      n33 = case shown="2" w93 {
        tunnel: w96 -> [w127 _ _]
        tunnel: w95 -> [_ _ w149]
        tunnel: w94 -> [w100 _ _]
        frame 0, Default {
          n34 = Unbundle By Name(w127) -> ("ECC"=w113:T10, "Barcode Polarity"=w112:T6, "Bounding Box"=w124:cluster{"x":sgl, "y":sgl}[], "Border Integrity"=w120:sgl, "Aspect Ratio"=w108:sgl, "Minimum Edge Strength"=w118:u32, "Cell Fill Percentage"=w106:T11, "Demodulation Mode"=w105:T2, "Cell Sample Size"=w104:T3, "Cell Filter Mode"=w103:T4, "Mirrored?"=w123:bool)
          n35 = for {
            tunnel: T15[] [{"Option"=enum."Line Detection", " Value"=0.0}, {"Option"=enum."HighLight Filter", " Value"=0.0}, {"Option"=enum."Aggressive", " Value"=0.0}, {"Option"=enum."FNC1", " Value"=0.0}, {"Option"=enum."Refine Bounding Box", " Value"=0.0}] ("Advanced Options") -> [w133] mode=indexing
            tunnel: w100 -> [w132] mode=indexing
            tunnel: [w131] -> w99 mode=indexing
            n36 = Bundle By Name(cluster=w133, "Value"=w132) -> (w131:T15)
          }
          n37 = call "IMAQ Point Distances"("Points"=w124) -> ("Distances"=w126:sgl[], "error out"=w97:errorcluster)  [unwired: 1 in, 3 out]
          n38 = Subtract(x=w120, y=sgl 10.0) -> (x-y=w129:sgl)
          n39 = Boolean To (0,1)(Boolean=w123) -> (0, 1=w102:i16)
          n40 = To Unsigned Long Integer(number=w126) -> (unsigned 32bit integer=w125:u32[])
          n41 = In Range and Coerce(upper limit=sgl 100.0 ("lower limit"), x=w129, lower limit=sgl 80.0) -> (coerced(x)=w109:sgl)  [unwired: 1 out]
          n42 = Array Max & Min(array=w125) -> (max value=w122:u32, min value=w121:u32)  [unwired: 2 out]
          n43 = call <vilib>:"Clear Errors.vi"("error in (no error)"=w97) -> ()  [unwired: 5 in, 2 out]
          n44 = Multiply(x=w122, y=1.1) -> (x*y=w110:dbl)
          n45 = Multiply(x=w121, y=0.9) -> (x*y=w111:dbl)
          n46 = Multiply(x=w118, y=sgl 0.9 ("x")) -> (x*y=w107:sgl)
          n47 = Bundle By Name(cluster=T16 {"Data Matrix Description Options"={"Aspect Ratio"=0.0, "Rows"=0, "Columns"=0, "Rectangle"=FALSE, "ECC"=-2, "Barcode Polarity"=-2, "Cell Fill Percentage"=-2, "Minimum Border Integrity %"=80.0, "Mirror Mode"=-2}, "Data Matrix Search Options"={"Rotation Mode"=enum."Unlimited", "Skip Location?"=FALSE, "Edge Threshold"=30, "Demodulation Mode"=-2, "Cell Sample Size"=-2, "Cell Filter Mode"=2, "Skew Degrees Allowed"=5, "Maximum Iterations"=100, "Initial Search Vector Width"=5}, "Data Matrix Size Options"={"Data Matrix Size"={"Minimum Size"=0, "Maximum Size"=0}, "Quiet Zone Width"=0}, "Advanced Options"=[]} ("Data Matrix Auto Detect Values Out"), "Advanced Options"=w99, "Data Matrix Description Options.ECC"=w113, "Data Matrix Description Options.Barcode Polarity"=w112, "Data Matrix Size Options.Data Matrix Size.Minimum Size"=w111, "Data Matrix Size Options.Data Matrix Size.Maximum Size"=w110, "Data Matrix Description Options.Minimum Border Integrity %"=w109, "Data Matrix Description Options.Aspect Ratio"=w108, "Data Matrix Search Options.Edge Threshold"=w107, "Data Matrix Description Options.Cell Fill Percentage"=w106, "Data Matrix Search Options.Demodulation Mode"=w105, "Data Matrix Search Options.Cell Sample Size"=w104, "Data Matrix Search Options.Cell Filter Mode"=w103, "Data Matrix Description Options.Mirror Mode"=w102) -> (→"Data Matrix Auto Detect Values Out":T16)
        }
        frame 1 {
        }
        frame 2 {
          w147 = sgl 15.0 ("Auto Detect Value")
          w148 = sgl 3.0 ("Auto Detect Value")
          n48 = Unbundle By Name(w149) -> ("QR Model"=w145:T7, "Dimensions (Rows/Cols)"=w144:u32, "Barcode Polarity"=w143:T6, "Bounding Box"=w162:cluster{"x":sgl, "y":sgl}[], "Minimum Edge Strength"=w159:u32, "Demodulation Mode"=w139:T2, "Cell Sample Size"=w138:T3, "Cell Filter Mode"=w137:T4, "Mirrored?"=w157:bool)
          n49 = call "IMAQ Point Distances"("Points"=w162) -> ("Distances"=w166:sgl[], "error out"=w134:errorcluster)  [unwired: 1 in, 3 out]
          n50 = Equal To 0?(x=w145) -> (x = 0?=w154:bool)
          n51 = To Unsigned Long Integer(number=w166) -> (unsigned 32bit integer=w165:u32[])
          n52 = Array Max & Min(array=w165) -> (max value=w164:u32, min value=w163:u32)  [unwired: 2 out]
          n53 = call <vilib>:"Clear Errors.vi"("error in (no error)"=w134) -> ()  [unwired: 5 in, 2 out]
          n54 = Boolean To (0,1)(Boolean=w157) -> (0, 1=w136:i16)
          n55 = Divide(x=w159, y=u32 2) -> (x/y=w140:dbl)
          n56 = Multiply(x=w164, y=1.5) -> (x*y=w156:dbl)
          n57 = Multiply(x=w163, y=0.5) -> (x*y=w155:dbl)
          n58 = Divide(x=w156, y=w144) -> (x/y=w153:dbl)
          n59 = Divide(x=w155, y=w144) -> (x/y=w151:dbl)
          n60 = Max & Min(x=w151, y=w148) -> (max(x,y)=w150:dbl)  [unwired: 1 out]
          n61 = Max & Min(x=w153, y=w147) -> (min(x,y)=w152:dbl)  [unwired: 1 out]
          n62 = Select(t=w147, s=w154, f=w152) -> (s? t:f=w141:dbl)
          n63 = Select(t=w148, s=w154, f=w150) -> (s? t:f=w142:dbl)
          n64 = Bundle By Name(cluster=T8 {"QR Search Options"={"Rotation Mode"=enum."Unlimited", "Skip Location?"=FALSE, "Edge Threshold"=30, "Demodulation Mode"=-2, "Cell Sample Size"=-2, "Cell Filter Mode"=2, "Skew Degrees Allowed"=5}, "QR Description Options"={"Matrix Size (cells)"=0, "Barcode Polarity"=-2, "Mirror Mode"=-2, "QR Model"=0}, "QR Code Cell Size (pixels)"={"Minimum Size"=3, "Maximum Size"=15}} ("QR Code Auto Detect Values"), "QR Description Options.QR Model"=w145, "QR Description Options.Matrix Size (cells)"=w144, "QR Description Options.Barcode Polarity"=w143, "QR Code Cell Size (pixels).Minimum Size"=w142, "QR Code Cell Size (pixels).Maximum Size"=w141, "QR Search Options.Edge Threshold"=w140, "QR Search Options.Demodulation Mode"=w139, "QR Search Options.Cell Sample Size"=w138, "QR Search Options.Cell Filter Mode"=w137, "QR Description Options.Mirror Mode"=w136) -> (→"QR Code Auto Detect Values":T8)
        }
      }
    }
  }
